vi "Event Write.vi"(4 "error in (no error)":errorcluster, 5 "Value":refnum<user-event>, 6 "Container State":T3, 7 "Display State In":T1={"Cells_VD2"=enum."5", "position"=0.0, "DS param"={"Domain name"="manip", "experiment"="VD2", "Device Server name"="DLs_VD2", "DL param"={"real pos"=-137.0, "max"=-30.0, "min"=120.0}, "preset pos"=[-48.0, -24.0, 0.0, 24.0, 48.0]}, "event"=refnum}) -> (0 "error out":errorcluster, 3 "Display State Out":T1={"Cells_VD2"=enum."5", "position"=0.0, "DS param"={"Domain name"="manip", "experiment"="VD2", "Device Server name"="DLs_VD2", "DL param"={"real pos"=-137.0, "max"=-30.0, "min"=120.0}, "preset pos"=[-48.0, -24.0, 0.0, 24.0, 48.0]}, "event"=refnum})   [LabVIEW 2020, in "OWIS_DLs_h.xctl"]
uses:
  OWIS_DLs_h.xctl
  <vilib>/_xctls/Container State.ctl
  stateDL.ctl
  controls/CellsSDI.ctl
  controls/CellBoolean.ctl
  <vilib>/_xctls/XControlSupport.lvlib
panel:
  # "Replace the Value Control below with a Control of desired type.\nDo not remove this Control or the others from the connector pane.\nDo not change the connector pane pattern.\nThe Value control should always be the third terminal from top on the input side in the connector pane."
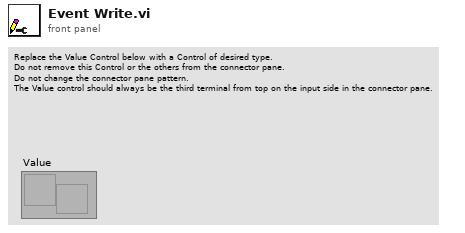
[diagram p1: front panel]
types:
  T1 = typedef "OWIS_DLs_h.xctl/stateDL.ctl" = cluster{"Cells_VD2":T2, "position":dbl, "DS param":cluster{"Domain name":string, "experiment":string, "Device Server name":string, "DL param":cluster{"real pos":dbl, "max":dbl, "min":dbl}, "preset pos":dbl[]}, "event":refnum<user-event>}
  T2 = typedef "CellsSDI.ctl" = enum32{"5", "4", "3", "2", "1", "L"}
  T3 = typedef "XControlSupport.lvlib/Container State.ctl" = cluster{"Indicator?":bool, "Run Mode?":bool, " Refnum":refnum<vi>}
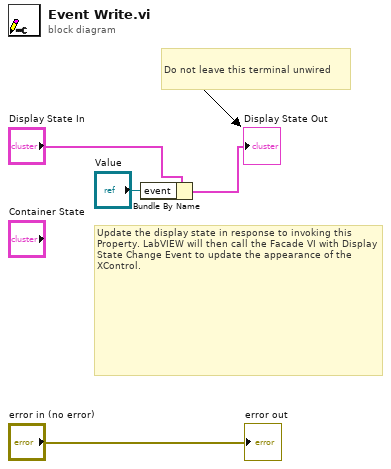
[diagram p0: block diagram]
diagram:
  # "Do not leave this terminal unwired"
  # "Update the display state in response to invoking this Property. LabVIEW will then call the Facade VI with Display State Change Event to update the appearance of the XControl."
  n1 = Bundle By Name(cluster="Display State In", "event"="Value") -> (→"Display State Out":T1)
  "error out" <- "error in (no error)"
